vi "state history.vi"(1 "command":enum16{"write", "read", "reset"}(ring), 2 "Plant State":T1=1 items=["OFF"], 3 "Time":dbl format="%.2f") -> (0 "state history":cluster{dbl[], T1[]} {"?" items=["OFF"]; "?" format="%.2f"})   [LabVIEW 2012]
uses:
  Plant state.ctl
  DAQ configuration/Sensor buffer command.ctl
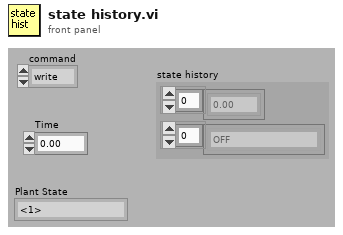
[diagram p1: front panel]
types:
  T1 = typedef "Plant state.ctl" = u16
  T2 = typedef "Sensor buffer command.ctl" = enum16{"read average", "read recent", "read all", "write", "configure", "clear"}
  T3 = typedef "Sensor data.ctl" = cluster{" Sensor array":T4[], "Time":dbl}
  T4 = typedef "sensor cluster.ctl" = cluster{"voltage":sgl, "scaled":sgl, "units":string, "Out of Range":bool}
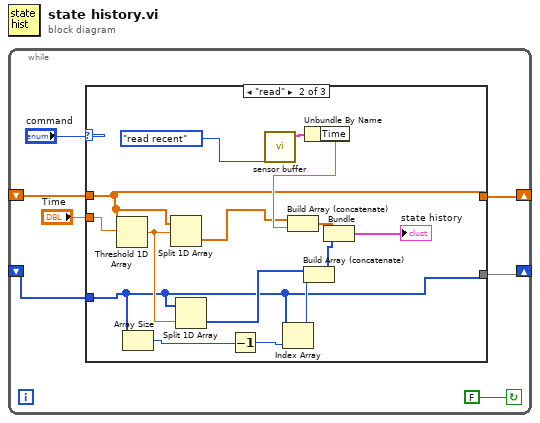
[diagram p0: block diagram]
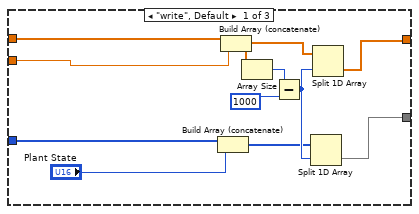
[diagram p2: hidden frame]
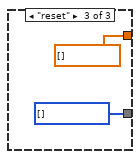
[diagram p3: hidden frame]
diagram:
  n1 = while {
    shift-right: [w5] -> _
    shift-left: _ -> [w4]
    shift-right: [w2] -> _
    shift-left: _ -> [w3]
    stop <- FALSE continue-if-true
    n2 = case shown="\"read\"" "command" {
      tunnel: [w17 w23 dbl[] []] -> w5
      tunnel: w4 -> [w18 w23 _]
      tunnel: w3 -> [w13 w20 _]
      tunnel: [w9 w20 w34] -> w2
      tunnel: "Time" -> [w8 w25 _]
      frame "write", Default {
        n3 = Build Array (concatenate)(w13, "Plant State") -> (w10:T1[])
        n4 = Build Array (concatenate)(w18, w8) -> (w16:dbl[])
        n5 = Array Size(array=w16) -> (size(s)=w15:i32)
        n6 = Subtract(x=w15, y=1000) -> (x-y=w11:i32)
        n7 = Split 1D Array(array=w10, index=w11) -> (second subarray=w9:T1[])  [unwired: 1 out]
        n8 = Split 1D Array(array=w16, index=w11) -> (second subarray=w17:dbl[])  [unwired: 1 out]
      }
      frame "read" {
        n9 = Threshold 1D Array(2:w25, 3:w23) -> (0:w22:dbl)  [unwired: 1 in]
        n10 = Array Size(array=w20) -> (size(s)=w32:i32)
        n11 = Split 1D Array(array=w23, index=w22) -> (second subarray=w24:dbl[])  [unwired: 1 out]
        n12 = Split 1D Array(array=w20, index=w22) -> (second subarray=w21:T1[])  [unwired: 1 out]
        n13 = Decrement(x=w32) -> (x-1=w31:i32)
        n14 = call "sensor buffer.vi"("command"=Sensor_buffer_command."read recent") -> ("Sensor Data smoothed"=w28:T3)  [unwired: 4 in, 2 out]
        n15 = Index Array(array=w20, index=w31) -> (element=w30:T1)
        n16 = Build Array (concatenate)(w21, w30) -> (w29:T1[])
        n17 = Unbundle By Name(w28) -> ("Time"=w27:dbl)
        n18 = Build Array (concatenate)(w24, w27) -> (w26:dbl[])
        n19 = Bundle(w26, w29) -> (→"state history":cluster{dbl[], T1[]})  [unwired: 1 in]
      }
      frame "reset" {
        w34 = T1[] [] items=["OFF"]
      }
    }
  }
